vi "Start Acquisition.vi"(8 "error in (no error)":errorcluster, 9 "Image Type":T1=1 items=["Grayscale (U8)", "Grayscale (I16)", "Grayscale (SGL)", "Complex (CSG)", "RGB (U32)", "HSL (U32)", "RGB (U64)", "Grayscale (U16)"], 10 "Camera Name":T2, 11 "IMAQdx Cam Actor in":refnum<class "IMAQdx Cam Actor.lvclass">) -> (0 "error out":errorcluster, 3 "IMAQdx Cam Actor out":refnum<class "IMAQdx Cam Actor.lvclass">)   [LabVIEW 2014, in "IMAQdx Cam Actor.lvlib" / "IMAQdx Cam Actor.lvclass"]
uses:
  IMAQdx Cam Actor.lvclass
  <vilib>/userdefined/High Color/IMAQdx.ctl
  <vilib>/vision/driver/IMAQdx.llb/IMAQdx Camera Control Mode.ctl
  <vilib>/vision/driver/IMAQdx.llb/IMAQdx Acquisition Mode.ctl
  IMAQdx Cam Actor.lvclass/IMAQdx Cam Actor.ctl
  <vilib>/vision/driver/NI_Vision_Acquisition_Software.lvlib
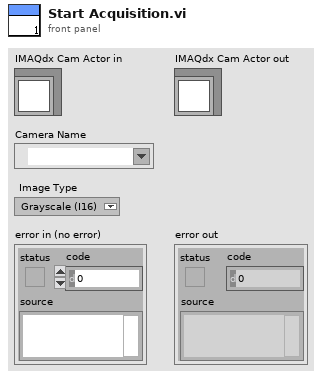
[diagram p1: front panel]
types:
  T1 = typedef "Image Type" = u32
  T2 = typedef "IMAQdx.ctl" = refnum<k21>
  T3 = typedef "NI_Vision_Acquisition_Software.lvlib/IMAQdx Acquisition Mode.ctl" = enum32{"One Shot", "Continuous"}
  T4 = typedef "NI_Vision_Acquisition_Software.lvlib/IMAQdx Camera Control Mode.ctl" = enum32{"Controller", "Listener"}
  T5 = typedef "IMAQ Image.ctl" = refnum<image>
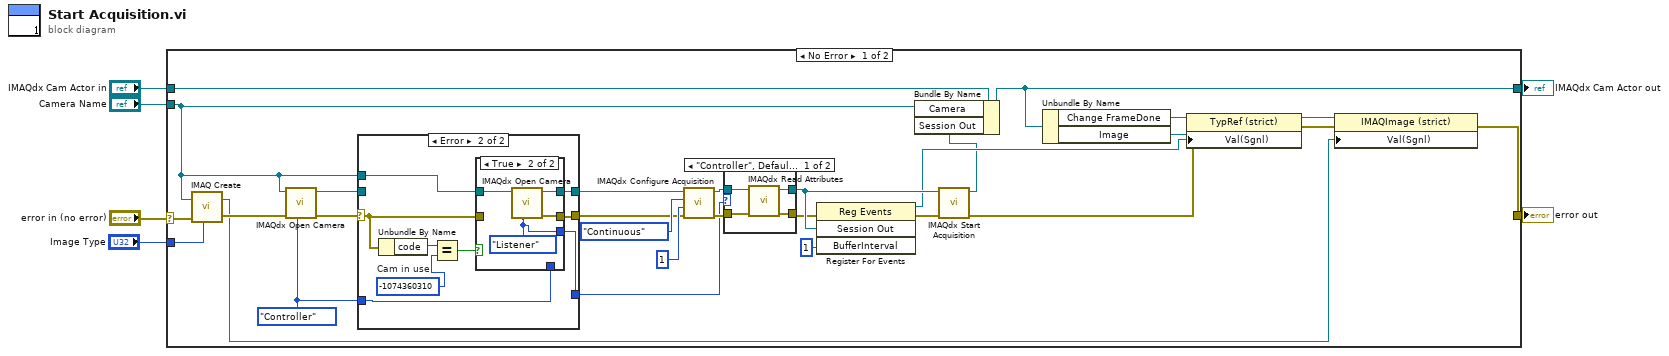
[diagram p0: block diagram]
diagram:
  n1 = case shown="No Error" "error in (no error)" {
    selector: "error in (no error)" -> [w19 w61]
    tunnel: [w7 w61] -> w5
    tunnel: [w14 w60] -> w3
    tunnel: "IMAQdx Cam Actor in" -> [w20 w60]
    tunnel: "Image Type" -> [w17 _]
    tunnel: "Camera Name" -> [w13 _]
    frame No Error {
      w22 = IMAQdx_Camera_Control_Mode."Controller" ("Camera Control Mode")
      n2 = call "IMAQ Create"("Image Name"=w13, "Image Type"=w17, "error in (no error)"=w19) -> ("New Image"=w10:T5, "error out"=w32:errorcluster)  [unwired: 1 in, 1 out]
      n3 = call <vilib>:"IMAQdx Open Camera.vi"("Camera Control Mode"=w22, "error in"=w32, "Session In"=w13) -> ("error out"=w30:errorcluster, "Session Out"=w34:T2)  [unwired: 7 out]
      n4 = case shown="Error" w30 {
        selector: w30 -> [w42 w47]
        tunnel: w34 -> [w43 _]
        tunnel: [w43 w50] -> w24
        tunnel: [w42 w49] -> w25
        tunnel: w13 -> [_ w46]
        tunnel: w22 -> [w41 w44]
        tunnel: [w41 w45] -> w21
        frame No Error {
        }
        frame Error {
          w51 = -1074360310  # Cam in use
          n5 = Unbundle By Name(w47) -> ("code"=w52:i32)
          n6 = Equal?(x=w52, y=w51) -> (x = y?=w48:bool)
          n7 = case shown="True" w48 {
            tunnel: w46 -> [w54 w59]
            tunnel: [w54 w57] -> w50
            tunnel: [w55 w58] -> w49
            tunnel: w47 -> [w55 _]
            tunnel: [w53 w56] -> w45
            tunnel: w44 -> [w53 _]
            frame False {
            }
            frame True {
              w56 = IMAQdx_Camera_Control_Mode."Listener" ("Camera Control Mode")
              n8 = call <vilib>:"IMAQdx Open Camera.vi"("Camera Control Mode"=w56, "Session In"=w59) -> ("error out"=w58:errorcluster, "Session Out"=w57:T2)  [unwired: 1 in, 7 out]
            }
          }
        }
      }
      n9 = call <vilib>:"IMAQdx Configure Acquisition.vi"("error in"=w25, "Number of Buffers"=u32 1, "Continuous?"=IMAQdx_Acquisition_Mode."Continuous", "Session In"=w24) -> ("error out"=w29:errorcluster, "Session Out"=w28:T2)  [unwired: 6 out]
      n10 = case shown="\"Controller\", Default" w21 {
        tunnel: w29 -> [w38 w39]
        tunnel: w28 -> [w37 w40]
        tunnel: [w36 w39] -> w18
        tunnel: [w35 w40] -> w23
        frame "Controller", Default {
          n11 = call <vilib>:"IMAQdx Read Attributes.vi"("error in"=w38, "Session In"=w37) -> ("error out"=w36:errorcluster, "Session Out"=w35:T2)  [unwired: 8 in]
        }
        frame "Listener" {
        }
      }
      n12 = register-events(error in=w18, w23, u32 1 ("BufferInterval")) -> (reference out=w15:refnum<event-registration>, error out=w33:errorcluster)  [unwired: 1 in]
      n13 = call <vilib>:"IMAQdx Start Acquisition.vi"("error in"=w33, "Session In"=w23) -> ("error out"=w8:errorcluster, "Session Out"=w12:T2)  [unwired: 8 out]
      n14 = Bundle By Name(cluster=w20, "Camera"=w13, "Session Out"=w12) -> (w14:refnum<class "IMAQdx Cam Actor.lvclass">)
      n15 = Unbundle By Name(w14) -> ("Change FrameDone"=w16:refnum<vi>, "Image"=w11:refnum<vi>)
      n16 = property class="TypRef (strict)"(reference=w16, error in=w8, "Val(Sgnl)"=w15) -> (error out=w9:errorcluster)  [unwired: 1 out]
      n17 = property class="IMAQImage (strict)"(reference=w11, error in=w9, "Val(Sgnl)"=w10) -> (error out=w7:errorcluster)  [unwired: 1 out]
    }
    frame Error {
    }
  }
  "error out" <- w5
  "IMAQdx Cam Actor out" <- w3
